vi "Example Simple.vi"() -> ()   [LabVIEW 2010]
uses:
  C:/tf/play/labview/Tinkerforge.dll
  Tinkerforge.dll
panel:
  out "distance (cm)":i32
  in  "uid":string="amb"
  in  "port":i32=4223
  in  "host":string="localhost"
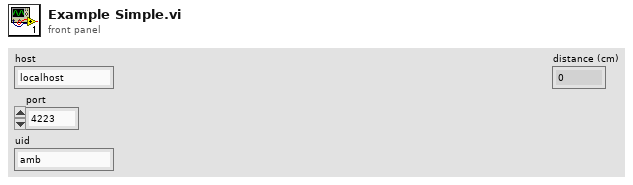
[diagram p1: front panel]
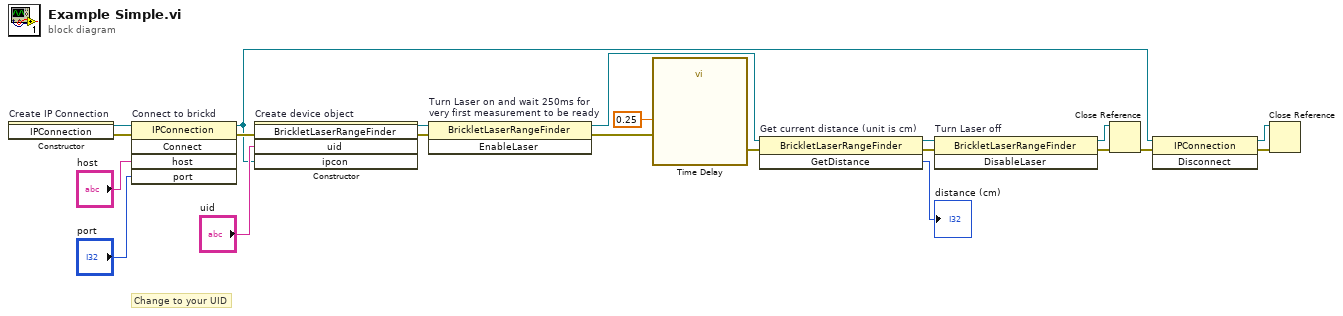
[diagram p0: block diagram]
diagram:
  # "Change to your UID"
  n1 = constructor on="Create IP Connection" class="IPConnection"() -> (reference out=w21:refnum<k24>, error out=w12:errorcluster)  [unwired: 3 in, 1 out]
  n2 = invoke on="Connect to brickd" class="IPConnection" method="Connect"(reference=w21, error in=w12, "host"="host", "port"="port") -> (reference out=w14:refnum<k24>, error out=w17:errorcluster)  [unwired: 1 in, 3 out]
  n3 = constructor on="Create device object" class="BrickletLaserRangeFinder"(error in=w17, "uid"="uid", "ipcon"=w14) -> (reference out=w5:refnum<k24>, error out=w6:errorcluster)  [unwired: 2 in, 3 out]
  n4 = invoke on="Turn Laser on and wait 250ms for\nvery first measurement to be ready" class="BrickletLaserRangeFinder" method="EnableLaser"(reference=w5, error in=w6) -> (reference out=w4:refnum<k24>, error out=w2:errorcluster)  [unwired: 1 in, 1 out]
  n5 = call "Time Delay"("error in (no error)"=w2, "Delay Time (s)"=0.25) -> ("error out"=w1:errorcluster)  [unwired: 9 in]
  n6 = invoke on="Get current distance (unit is cm)" class="BrickletLaserRangeFinder" method="GetDistance"(reference=w4, error in=w1) -> (reference out=w9:refnum<k24>, error out=w10:errorcluster, "GetDistance"=→"distance (cm)":i32)  [unwired: 1 in]
  n7 = invoke on="Turn Laser off" class="BrickletLaserRangeFinder" method="DisableLaser"(reference=w9, error in=w10) -> (reference out=w8:refnum<k24>, error out=w7:errorcluster)  [unwired: 1 in, 1 out]
  n8 = Close Reference(reference=w8, error in (no error)=w7) -> (error out=w16:errorcluster)
  n9 = invoke class="IPConnection" method="Disconnect"(reference=w14, error in=w16) -> (reference out=w13:refnum<k24>, error out=w15:errorcluster)  [unwired: 1 in, 1 out]
  n10 = Close Reference(reference=w13, error in (no error)=w15) -> ()  [unwired: 1 out]
